vi "EnviarParametros.vi"(0 "VISA resource name":refnum<visa-resource-name>, 5 "PASOS EN X":i32, 7 "PASOS EN Y":i32, 9 "PASOS EN Z":i32, 11 "error in (no error)":errorcluster) -> (4 "VISA resource name 2":refnum<visa-resource-name>, 15 "error out":errorcluster)   [LabVIEW 2019]
uses:
  <vilib>/Utility/error.llb/Error Cluster From Error Code.vi
  <vilib>/ErrorRing/Error Ring.xnode
panel:
  out "read buffer 2":string
  out "Parametros enviados = Parametros leídos? 2":bool
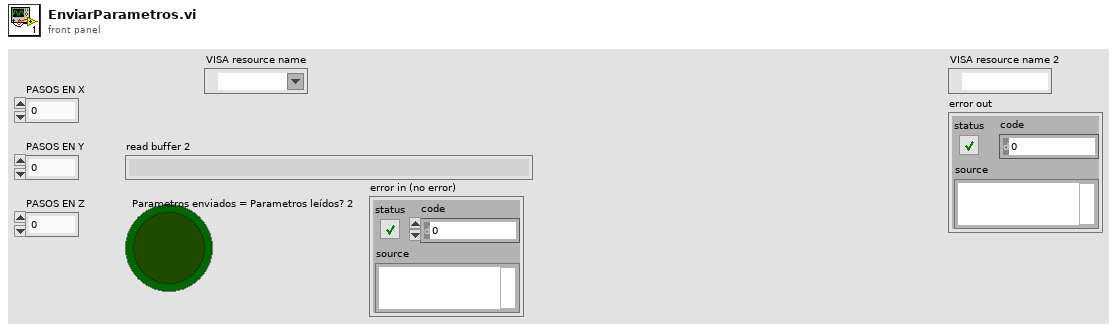
[diagram p1: front panel]
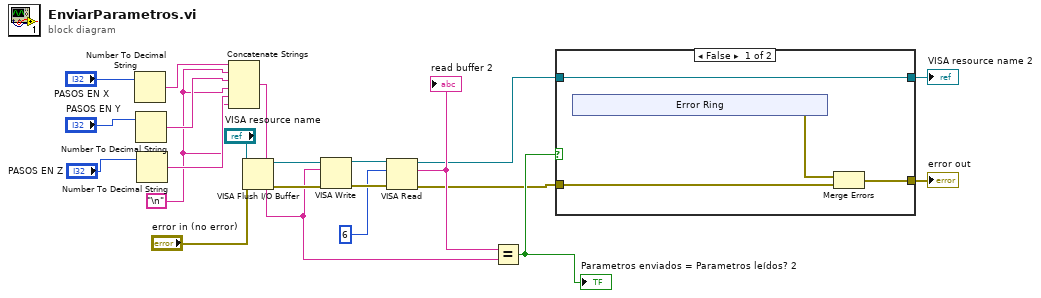
[diagram p0: block diagram]
diagram:
  w3 = "\n"
  n1 = Number To Decimal String(number="PASOS EN X") -> (decimal integer string=w13:string)  [unwired: 1 in]
  n2 = Number To Decimal String(number="PASOS EN Y") -> (decimal integer string=w14:string)  [unwired: 1 in]
  n3 = Number To Decimal String(number="PASOS EN Z") -> (decimal integer string=w15:string)  [unwired: 1 in]
  n4 = Concatenate Strings(w13, w3, w14, w3, w15, w3) -> (w1:string)
  n5 = VISA Flush I/O Buffer(VISA resource name="VISA resource name", error in (no error)="error in (no error)") -> (VISA resource name out=w12:refnum<visa-resource-name>, error out=w11:errorcluster)  [unwired: 1 in]
  n6 = VISA Write(VISA resource name=w12, write buffer=w1, error in (no error)=w11) -> (VISA resource name out=w20:refnum<visa-resource-name>, error out=w21:errorcluster)  [unwired: 1 out]
  n7 = VISA Read(VISA resource name=w20, byte count=u32 6, error in (no error)=w21) -> (VISA resource name out=w17:refnum<visa-resource-name>, read buffer=w19:string, error out=w16:errorcluster)  [unwired: 1 out]
  "read buffer 2" <- w19
  n8 = Equal?(x=w19, y=w1) -> (x = y?=w18:bool)
  "Parametros enviados = Parametros leídos? 2" <- w18
  n9 = case shown="False" w18 {
    tunnel: w16 -> [w24 w31]
    tunnel: [w23 w31] -> w4
    tunnel: w17 -> [w22 w32]
    tunnel: [w22 w32] -> w5
    frame False {
      n10 = xnode "Error Ring"() -> ("error out"=w25:errorcluster)
      n11 = Merge Errors(w25, w24) -> (w23:errorcluster)
    }
    frame True {
    }
  }
  "VISA resource name 2" <- w5
  "error out" <- w4
